vi "Session Cookie Name.vi"(8 "error in (no error)":errorcluster, 10 "Session Cookie Name":string, 11 "Server in":refnum<class "Server.lvclass">) -> (0 "error out":errorcluster, 3 "Server out":refnum<class "Server.lvclass">)   [LabVIEW 2020, in "HTTP Server.lvlib" / "Server.lvclass"]
uses:
  Server.lvclass
  Server.lvclass/Server.ctl
  Session/Session.lvclass
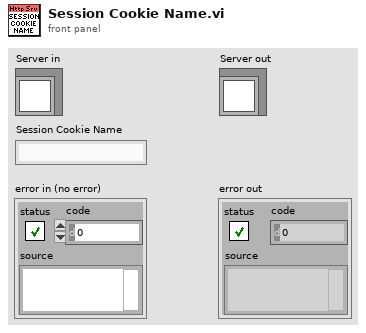
[diagram p1: front panel]
types:
  T1 = typedef "HTTP Server.lvlib/Server.lvclass/Ref Data.ctl" = cluster{"Connection Handler Map":T2, "Request Handler Map":T4, "Route Handler Map":T5, "Controller Handler Map":T6, "Controller Map":T7, "Response Handler Map":T8, "Complete Handler Map":T9, "Exception Handler Map":T10, "Connection Handler Index":u16, "Request Handler Index":u16, "Route Handler Index":u16, "Controller Handler Index":u16, "Controller Index":u16, "Response Handler Index":u16, "Complete Handler Index":u16, "Exception Handler Index":u16, "Values":refnum<class "Values.lvclass">, "Path":path, "Session Type":refnum<class "Session.lvclass">, "Session Cookie Name":string, "WebSocket Handler":refnum<class "WebSocket Handler.lvclass">, "WebSocket Handling":bool}
  T2 = typedef "HTTP Server.lvlib/Connection Handler Map.ctl" = map{T3, refnum<class "Connection Handler.lvclass">}
  T3 = typedef "HTTP Server.lvlib/Priority.ctl" = cluster{"Entity":u16, "Index":u16}
  T4 = typedef "HTTP Server.lvlib/Request Handler Map.ctl" = map{T3, refnum<class "Request Handler.lvclass">}
  T5 = typedef "HTTP Server.lvlib/Route Handler Map.ctl" = map{T3, refnum<class "Route Handler.lvclass">}
  T6 = typedef "HTTP Server.lvlib/Controller Handler Map.ctl" = map{T3, refnum<class "Controller Handler.lvclass">}
  T7 = typedef "HTTP Server.lvlib/Controller Map.ctl" = map{T3, refnum<class "Controller.lvclass">}
  T8 = typedef "HTTP Server.lvlib/Response Handler Map.ctl" = map{T3, refnum<class "Response Handler.lvclass">}
  T9 = typedef "HTTP Server.lvlib/Complete Handler Map.ctl" = map{T3, refnum<class "Complete Handler.lvclass">}
  T10 = typedef "HTTP Server.lvlib/Exception Handler Map.ctl" = map{T3, refnum<class "Exception Handler.lvclass">}
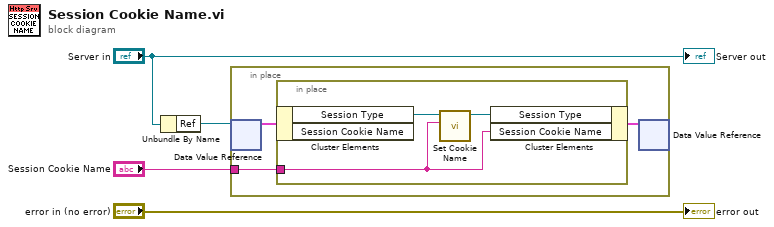
[diagram p0: block diagram]
diagram:
  n1 = Unbundle By Name("Server in") -> ("Ref"=w3:refnum<data-value>)
  n2 = in-place {
    in-place-border: "Session Cookie Name" -> [w5]
    n3 = in-place-dvr #1(w3) -> (w7:T1)  [unwired: 1 out]
    n4 = in-place {
      in-place-border: w5 -> [w8]
      n5 = in-place-cluster #2(w7) -> ("Session Type"=w10:refnum<class "Session.lvclass">)  [unwired: 1 out]
      n6 = call "Set Cookie Name.vi"("Cookie Name"=w8, "Session in"=w10) -> ("Session out"=w9:refnum<class "Session.lvclass">)  [unwired: 8 in, 1 out]
      n7 = in-place-cluster #2("Session Type"=w9, "Session Cookie Name"=w8) -> (w6:T1)
    }
    n8 = in-place-dvr #1(w6) -> ()  [unwired: 2 out]
  }
  "error out" <- "error in (no error)"
  "Server out" <- "Server in"
